vi "MotionProfiling_2D_PushPoint.vi"(7 "Motion Profile Status":T6, 8 "CursorIn":i32, 9 "NumberOfPoints":i32, 10 "ArrayOfTrajectoyPoints":dbl[][](array[numeric]), 11 "PhoenixMotorControlDevRef":T1={"DeviceStatus"={"status"=FALSE, "code"=0, "source"=""}, "Type"=enum."PWM", "PWM"={"PWM Channel"=enum."Invalid", "DeadBand"={"Name"="", "maxPositivePwm"=0, "minPositivePwm"=0, "centerPwm"=0, "maxNegativePwm"=0, "minNegativePwm"=0, "angularRange"=0}}, "CAN"={"Device Number"=0, "SetOutput VI Ref"=variant, "GetOutput VI Ref"=variant, "Enable VI Ref"=variant, "Disable VI Ref"=variant, "Data"=variant}, "Invert"=FALSE, "DIO PWM"={"PWM \"Enable\" Channel"=enum."Invalid", "DIOChannel"=enum."Invalid", "PWM Rate"=0.0}}) -> (0 "CursorOut":u32, 3 "PhoenixMotorControlDevRef Out":T1={"DeviceStatus"={"status"=FALSE, "code"=0, "source"=""}, "Type"=enum."PWM", "PWM"={"PWM Channel"=enum."Invalid", "DeadBand"={"Name"="", "maxPositivePwm"=0, "minPositivePwm"=0, "centerPwm"=0, "maxNegativePwm"=0, "minNegativePwm"=0, "angularRange"=0}}, "CAN"={"Device Number"=0, "SetOutput VI Ref"=variant, "GetOutput VI Ref"=variant, "Enable VI Ref"=variant, "Disable VI Ref"=variant, "Data"=variant}, "Invert"=FALSE, "DIO PWM"={"PWM \"Enable\" Channel"=enum."Invalid", "DIOChannel"=enum."Invalid", "PWM Rate"=0.0}})   [LabVIEW 2017]
uses:
  <vilib>/Rock Robotics/WPI/MotorControl/WPI_MotorControlDeviceRef.ctl
  <vilib>/Rock Robotics/WPI/MotorControl/WPI_MotorControlType.ctl
  <vilib>/Rock Robotics/SystemInterfaces/DIO/FPGA_DIOPWMChannel.ctl
  <vilib>/Rock Robotics/WPI/PWM/WPI_PWMDeadband.ctl
  <vilib>/Rock Robotics/SystemInterfaces/DIO/FPGA_DIOChannel.ctl
  <vilib>/Rock Robotics/WPI/ThirdParty/Phoenix-LabVIEW/Motor Controller/Controls/CTRE_Phoenix_MotorControl_TrajectoryPointTimeDur.ctl
panel:
  in  "Number of Encoder Ticks/ rotation":dbl=4096.0
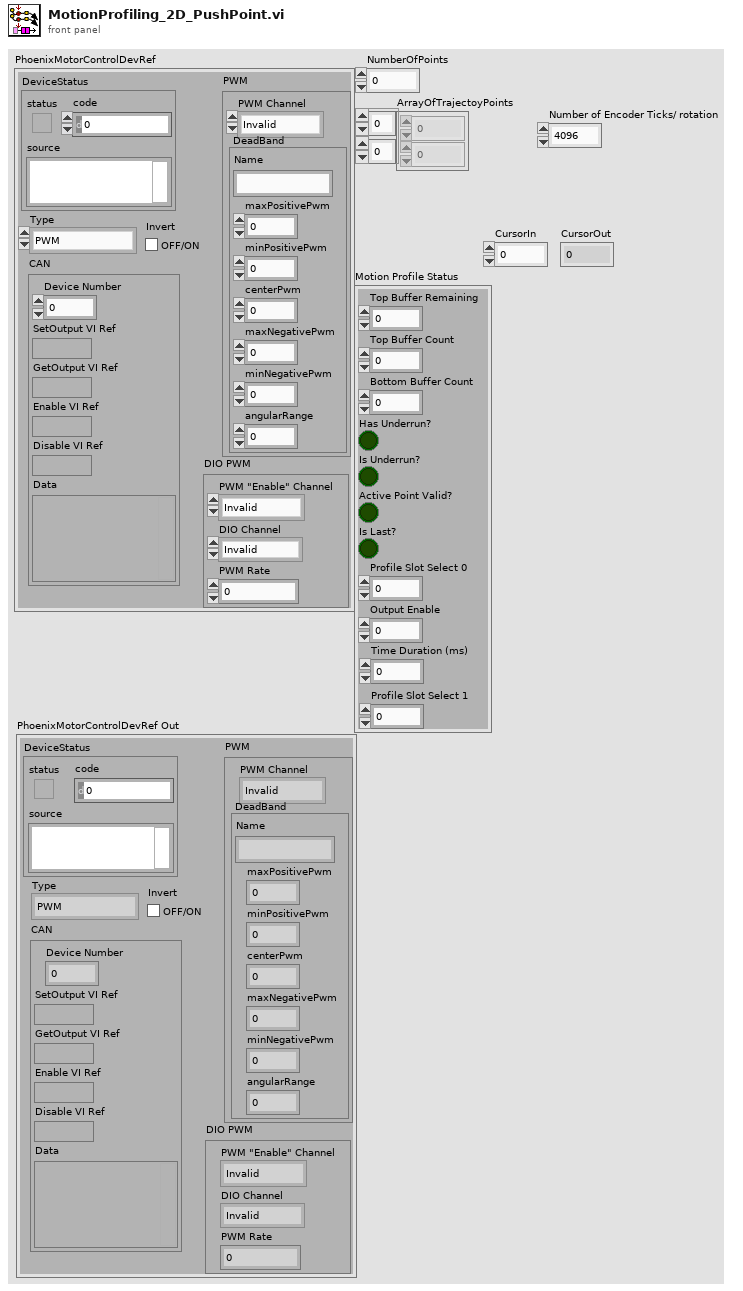
[diagram p1: front panel]
types:
  T1 = typedef "WPI_MotorControlDeviceRef.ctl" = cluster{"DeviceStatus":errorcluster, "Type":T2, "PWM":cluster{"PWM Channel":T3, "DeadBand":T4}, "CAN":cluster{"Device Number":u8, "SetOutput VI Ref":variant, "GetOutput VI Ref":variant, "Enable VI Ref":variant, "Disable VI Ref":variant, "Data":variant}, "Invert":bool, "DIO PWM":cluster{"PWM \"Enable\" Channel":T3, "DIOChannel":T5, "PWM Rate":dbl}}
  T2 = typedef "WPI_MotorControlType.ctl" = enum16{"PWM", "CAN", "DIO PWM"}
  T3 = typedef "FPGA_DIOPWMChannel.ctl" = enum8{"PWM 0", "PWM 1", "PWM 2", "PWM 3", "PWM 4", "PWM 5", "PWM 6", "PWM 7", "PWM 8", "PWM 9", "PWM MXP 0", "PWM MXP 1", "PWM MXP 2", "PWM MXP 3", "PWM MXP 4", "PWM MXP 5", "PWM MXP 6", "PWM MXP 7", "PWM MXP 8", "PWM MXP 9", "Invalid"}
  T4 = typedef "WPI_PWMDeadband.ctl" = cluster{"Name":string, "maxPositivePwm":i32, "minPositivePwm":i32, "centerPwm":i32, "maxNegativePwm":i32, "minNegativePwm":i32, "angularRange":u16}
  T5 = typedef "FPGA_DIOChannel.ctl" = enum8{"DIO 0", "DIO 1", "DIO 2", "DIO 3", "DIO 4", "DIO 5", "DIO 6", "DIO 7", "DIO 8", "DIO 9", "DIO MXP 0", "DIO MXP 1", "DIO MXP 2", "DIO MXP 3", "DIO MXP 4", "DIO MXP 5", "DIO MXP 6", "DIO MXP 7", "DIO MXP 8", "DIO MXP 9", "DIO MXP 10", "DIO MXP 11", "DIO MXP 12", "DIO MXP 13", "DIO MXP 14", "DIO MXP 15", "SPI Port CS1", "SPI Port CS2", "SPI Port CS3", "SPI Port MISO", "SPI Port MOSI", "Invalid"}
  T6 = cluster{"Top Buffer Remaining":i32, "Top Buffer Count":i32, "Bottom Buffer Count":i32, "Has Underrun?":bool, "Is Underrun?":bool, "Active Point Valid?":bool, "Is Last?":bool, "Profile Slot Select 0":i32, "Output Enable":i32, "Time Duration (ms)":i32, "Profile Slot Select 1":i32}
  T7 = typedef "CTRE_Phoenix_MotorControl_TrajectoryPointTimeDur.ctl" = i32
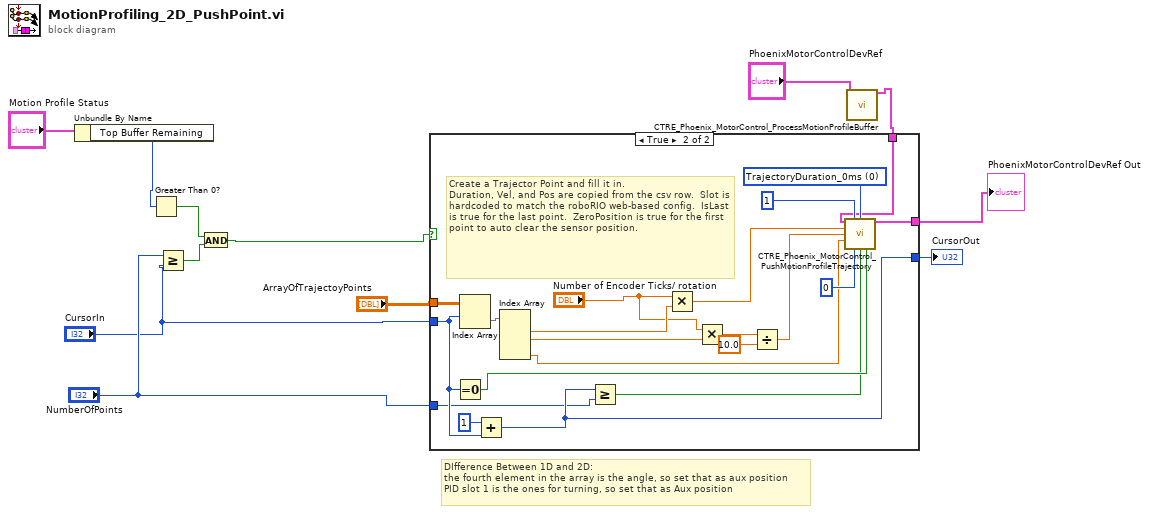
[diagram p0: block diagram]
diagram:
  # "DIfference Between 1D and 2D: \nthe fourth element in the array is the angle, so set that as aux position\nPID slot 1 is the ones for turning, so set that as Aux position"
  n1 = Unbundle By Name("Motion Profile Status") -> ("Top Buffer Remaining"=w4:i32)
  n2 = Greater Than 0?(x=w4) -> (x > 0?=w5:bool)
  n3 = Greater Or Equal?(x="NumberOfPoints", y="CursorIn") -> (x >= y?=w10:bool)
  n4 = And(x=w5, y=w10) -> (x .and. y?=w9:bool)
  n5 = call <vilib>:"CTRE_Phoenix_MotorControl_ProcessMotionProfileBuffer.vi"("PhoenixMotorControlDevRef"="PhoenixMotorControlDevRef") -> ("PhoenixMotorControlDevRef"=w2:T1)  [unwired: 13 in, 1 out]
  n6 = case shown="True" w9 {
    tunnel: "ArrayOfTrajectoyPoints" -> [_ w35]
    tunnel: [w14 w31] -> w12
    tunnel: "CursorIn" -> [w14 w32]
    tunnel: "NumberOfPoints" -> [_ w30]
    tunnel: w2 -> [w13 w18]
    tunnel: [w13 w16] -> w1
    frame False {
    }
    frame True {
      w20 = T7 0 items=["TrajectoryDuration_0ms"=0, "TrajectoryDuration_5ms"=5, "TrajectoryDuration_10ms"=10, "TrajectoryDuration_20ms"=20, "TrajectoryDuration_30ms"=30, "TrajectoryDuration_40ms"=40, "TrajectoryDuration_50ms"=50, "TrajectoryDuration_100ms"=100] ("durationMs")
      # "Create a Trajector Point and fill it in.\nDuration, Vel, and Pos are copied from the csv row.  Slot is hardcoded to match the roboRIO web-based config.  IsLast is true for the last point.  ZeroPosition is true for the first point to auto clear the sensor position."
      n7 = Equal To 0?(x=w32) -> (x = 0?=w28:bool)
      n8 = Index Array(array=w35, index (row)=w32) -> (element=w33:dbl[])  [unwired: 1 in]
      n9 = Add(x=u32 1, y=w32) -> (x+y=w31:u32)
      n10 = Index Array(array=w33) -> (element #1=w25:dbl, element #2=w23:dbl, element #4=w15:dbl)  [unwired: 4 in, 1 out]
      n11 = Greater Or Equal?(x=w31, y=w30) -> (x >= y?=w27:bool)
      n12 = Multiply(x="Number of Encoder Ticks/ rotation", y=w25) -> (x*y=w24:dbl)
      n13 = Multiply(x="Number of Encoder Ticks/ rotation", y=w23) -> (x*y=w22:dbl)
      n14 = Divide(x=w22, y=10.0) -> (x/y=w21:dbl)
      n15 = call <vilib>:"CTRE_Phoenix_MotorControl_PushMotionProfileTrajectory.vi"("PhoenixMotorControlDevRef"=w18, "profileSlotSelect1"=1, "durationMs"=w20, "position"=w24, "velocity"=w21, "auxiliaryPos"=w15, "profileSlotSelect0"=0, "isLastPoint?"=w27, "Zero Position?"=w28) -> ("PhoenixMotorControlDevRef"=w16:T1)  [unwired: 5 in, 1 out]
    }
  }
  "CursorOut" <- w12
  "PhoenixMotorControlDevRef Out" <- w1
